vi "PA Start Get Data.vi"(10 "Channel":i32, 11 "DevHandle":i32) -> (3 "function return":i32)   [LabVIEW 2010, in "power_analyzer.lvlib"]
doc: "int WINAPI PA_StartGetData(int DevHandle,int Channel);"
uses:
  power_analyzer.lvlib
  USB2XXX/trunk/USB2XXX/USB2XXX/vs2010/Release/USB2XXX.dll
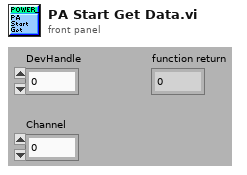
[diagram p1: front panel]
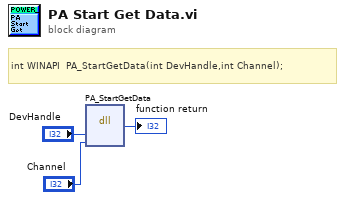
[diagram p0: block diagram]
diagram:
  # "int WINAPI  PA_StartGetData(int DevHandle,int Channel);"
  n1 = dll-call lib="E:/Projects/USB2XXX/trunk/USB2XXX/USB2XXX/vs2010/Release/USB2XXX.*" fn="PA_StartGetData"("DevHandle"="DevHandle", "Channel"="Channel") -> (→"function return":i32)  [unwired: 5 in, 2 out]
